vi "SubVI_activity4.vi"() -> ()   [LabVIEW 2025]
panel:
  out "Tank Volume":dbl(knob) scale=0.0..1000.0
  in  "Volume":bool
  # "Litters"
  # "Gallons"
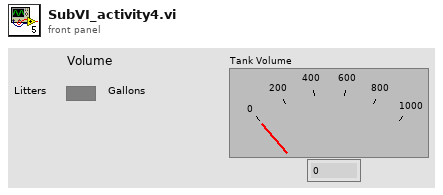
[diagram p1: front panel]
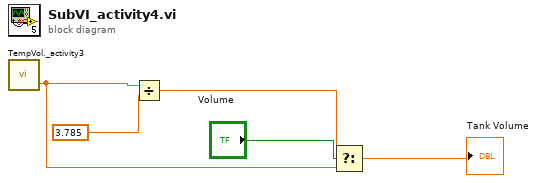
[diagram p0: block diagram]
diagram:
  n1 = call "TempVol._activity3.vi"() -> ("Volume"=w1:dbl)  [unwired: 1 out]
  n2 = Divide(x=w1, y=3.785) -> (x/y=w3:dbl)
  n3 = Select(t=w3, s="Volume", f=w1) -> (s? t:f=→"Tank Volume":dbl)
